vi "System_test.vi"() -> ()   [LabVIEW 2020]
panel:
  out "error out":errorcluster
  out "Button":bool
  in  "stop":bool
  in  "magnets":bool
  in  "Bolt right":bool
  in  "Bolt left":bool
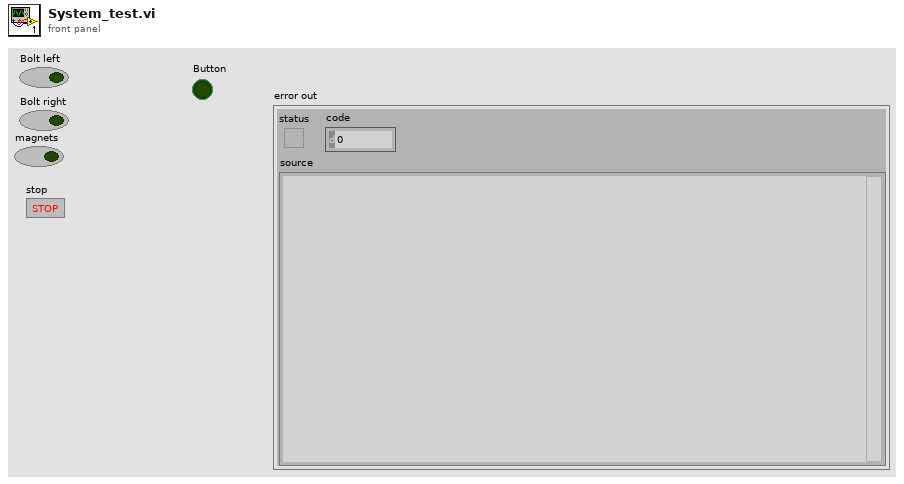
[diagram p1: front panel]
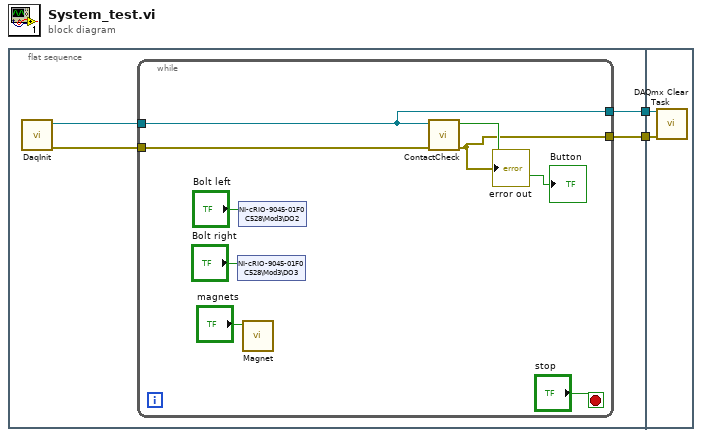
[diagram p0: block diagram]
diagram:
  n1 = flat-sequence {
    tunnel: [w4] -> w2
    tunnel: [w3] -> w1
    tunnel: w2 -> [w16]
    tunnel: w1 -> [w15]
    frame #0 {
      n2 = call "DaqInit.vi"() -> ("error out"=w6:errorcluster, "Refnum out"=w5:refnum<k21>)  [unwired: 10 in]
      n3 = while {
        tunnel: w6 -> [w10]
        tunnel: w5 -> [w9]
        tunnel: [w7] -> w4
        tunnel: [w9] -> w3
        stop <- "stop" stop-if-true
        n4 = shared-variable "NI-cRIO-9045-01F0C528\\Mod3\\DO3"("Bolt right") -> ()  [unwired: 1 in, 1 out]
        n5 = shared-variable "NI-cRIO-9045-01F0C528\\Mod3\\DO2"("Bolt left") -> ()  [unwired: 1 in, 1 out]
        n6 = call "Magnet.vi"("on_off"="magnets") -> ()  [unwired: 11 in]
        n7 = call "ContactCheck.vi"("error in"=w10, "task in"=w9) -> ("error out"=w7:errorcluster, "Boolesch"=→"Button":bool)  [unwired: 8 in]
        "error out" <- w7
      }
    }
    frame #1 {
      n8 = call <vilib>:"DAQmx Clear Task.vi"("task in"=w15, "error in"=w16) -> ()  [unwired: 13 in, 1 out]
    }
  }
